vi "Read Events.vi"(8 "error in (no error)":errorcluster, 11 "EST Digital Event in":refnum<class "Digital Event.lvclass">) -> (0 "error out":errorcluster, 2 "Events":u32, 3 "EST Digital Event out":refnum<class "Digital Event.lvclass">)   [LabVIEW 2019, in "Digital Event.lvclass"]
uses:
  Digital Event.lvclass
  Digital Event.lvclass/Digital Event.ctl
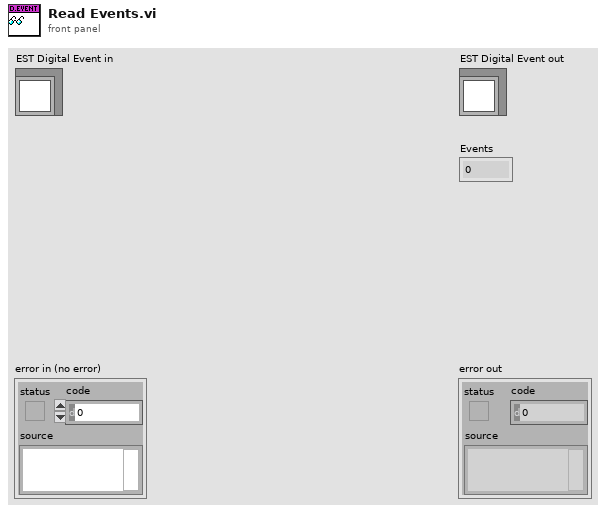
[diagram p1: front panel]
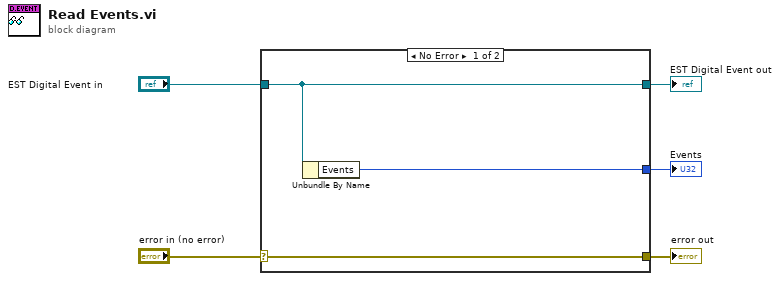
[diagram p0: block diagram]
diagram:
  n1 = case shown="No Error" "error in (no error)" {
    selector: "error in (no error)" -> [w8 w9]
    tunnel: [w8 w9] -> w4
    tunnel: [w7 w10] -> w2
    tunnel: "EST Digital Event in" -> [w7 w10]
    tunnel: [w6 _] -> w1
    frame No Error {
      n2 = Unbundle By Name(w7) -> ("Events"=w6:u32)
    }
    frame Error {
    }
  }
  "error out" <- w4
  "EST Digital Event out" <- w2
  "Events" <- w1
